vi "Generic Camera Get New Camera Image.vi"(0 "Camera Notifier Name":string, 13 "Frames":u16=1) -> (4 "Camera Notifier Name (Dup)":string, 8 "Image - U16":u16[][](array[numeric]), 15 "Error":errorcluster)   [LabVIEW 2025]
uses:
  Camera Controls/Generic Camera Actions.ctl
  Camera Controls/Camera IMAQ Key Info.ctl
panel:
  in  "Error In":errorcluster
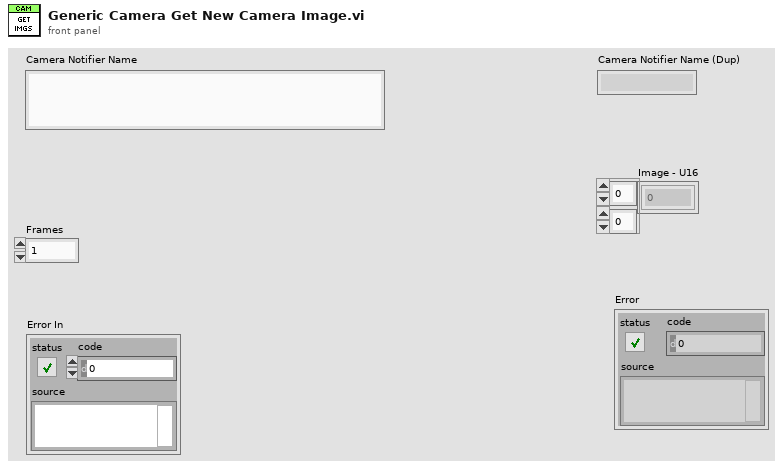
[diagram p1: front panel]
types:
  T1 = typedef "Generic Camera Actions.ctl" = enum16{"Status", "Live Preview", "Capture", "Abort", "Set Exposure Time (s)", "Get Exposure Time (s)", "Record Settings", "Binning", "Set ROI", "Get ROI", "Defect Correction On?", "Cooler On?", "Fan On?", "Quit"}
  T2 = typedef "IMAQ Image.ctl" = refnum<image>
  T3 = typedef "Camera IMAQ Key Info.ctl" = cluster{"Frame":u32, "Sensor Height":i32, "Sensor Width":i32, "ROI Height":i32, "ROI Width":i32, "ROI Enable?":bool, "Bit per Pixel":u8}
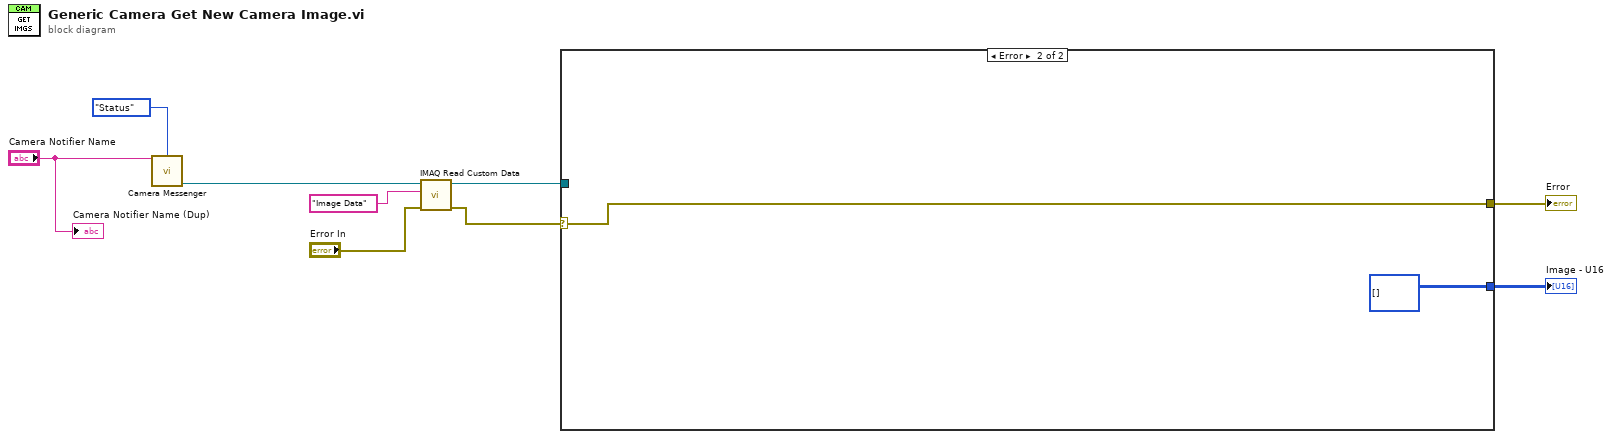
[diagram p0: block diagram]
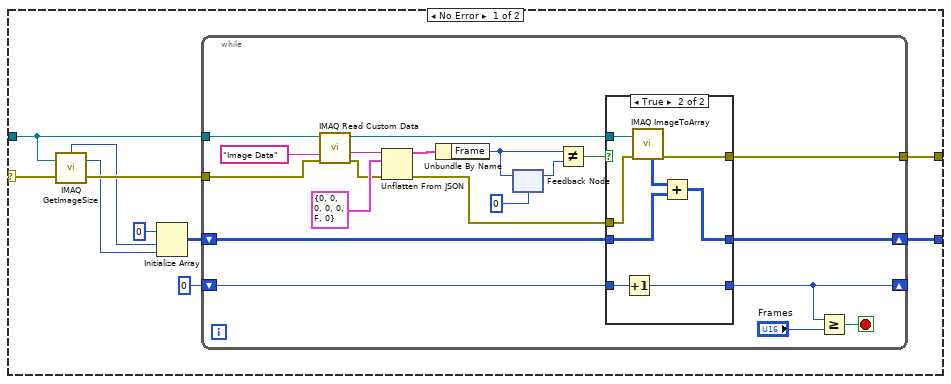
[diagram p2: hidden frame]
diagram:
  n1 = call "Camera Messenger.vi"("Notifier Name"="Camera Notifier Name", "General Camera Actions"=Generic_Camera_Actions."Status") -> ("Image Ref"=w5:T2)  [unwired: 8 in, 5 out]
  n2 = call "IMAQ Read Custom Data"("error in (no error)"="Error In", "Key"="Image Data", "Image"=w5) -> ("error out"=w1:errorcluster, "Image (duplicate)"=w4:T2)  [unwired: 6 in, 1 out]
  n3 = case shown="Error" w1 {
    selector: w1 -> [w10 w51]
    tunnel: w4 -> [w13 _]
    tunnel: [w16 w51] -> w9
    tunnel: [w15 u16[][] []] -> w8
    frame No Error {
      n4 = call "IMAQ GetImageSize"("Image"=w13, "error in (no error)"=w10) -> ("Y Resolution"=w12:i32, "X Resolution"=w11:i32, "error out"=w14:errorcluster)  [unwired: 2 in]
      n5 = Initialize Array(u16 0 ("element"), w11, w12) -> (w17:u16[][])
      n6 = while {
        shift-right: [w27] -> _
        shift-left: u16 0 -> [w28]
        shift-right: [w25] -> w15
        shift-left: w17 -> [w29]
        tunnel: w13 -> [w36]
        tunnel: w14 -> [w23]
        tunnel: [w20] -> w16
        stop <- w26 stop-if-true
        n7 = call "IMAQ Read Custom Data"("error in (no error)"=w23, "Key"="Image Data", "Image"=w36) -> ("error out"=w22:errorcluster, "Custom Data Out"=w38:string, "Image (duplicate)"=w30:T2)  [unwired: 6 in]
        n8 = Unflatten From JSON(JSON string=w38, type and defaults=T3 {"Frame"=0, "Sensor Height"=0, "Sensor Width"=0, "ROI Height"=0, "ROI Width"=0, "ROI Enable?"=FALSE, "Bit per Pixel"=0} ("Camera IMAQ Key Info"), error in (no error)=w22) -> (value=w35:T3, error out=w21:errorcluster)  [unwired: 4 in]
        n9 = Unbundle By Name(w35) -> ("Frame"=w33:u32)
        n10 = feedback-in #1(w33) -> ()
        n11 = feedback #1(u32 0) -> (w32:u32)
        n12 = Not Equal?(x=w33, y=w32) -> (x != y?=w31:bool)
        n13 = case shown="True" w31 {
          tunnel: w30 -> [_ w48]
          tunnel: w29 -> [w42 w47]
          tunnel: w28 -> [w41 w50]
          tunnel: [w41 w49] -> w27
          tunnel: [w42 w46] -> w25
          tunnel: w21 -> [w40 w45]
          tunnel: [w40 w44] -> w20
          frame False {
          }
          frame True {
            n14 = Increment(x=w50) -> (x+1=w49:u16)
            n15 = call "IMAQ ImageToArray"("error in (no error)"=w45, "Image"=w48) -> ("Image Pixels (U16)"=w43:u16[][], "error out"=w44:errorcluster)  [unwired: 2 in, 3 out]
            n16 = Add(x=w43, y=w47) -> (x+y=w46:u16[][])
          }
        }
        n17 = Greater Or Equal?(x=w27, y="Frames") -> (x >= y?=w26:bool)
      }
    }
    frame Error {
    }
  }
  "Error" <- w9
  "Image - U16" <- w8
  "Camera Notifier Name (Dup)" <- "Camera Notifier Name"
